vi "Color class 3 sect.vi"(7 "error in":errorcluster) -> (27 "error out":errorcluster)   [LabVIEW 2020]
uses:
  <vilib>/vision/Classification.llb/IMAQ Classifier Read Options.ctl
  <vilib>/vision/NI_Vision_Development_Module.lvlib
panel:
  out "Image Out":T1(plugin-control)
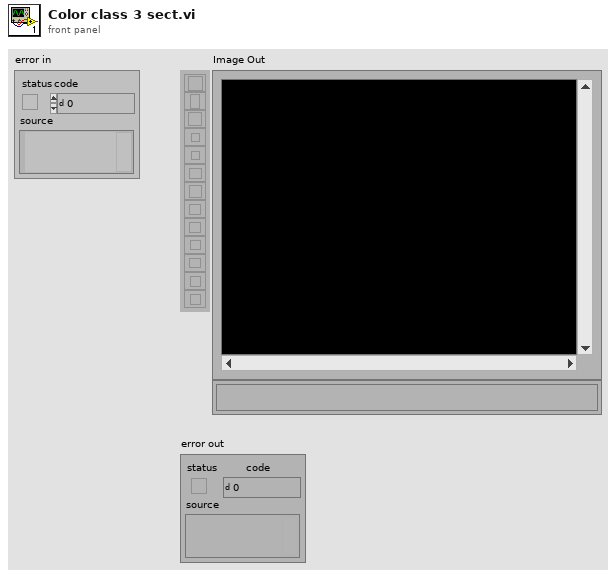
[diagram p1: front panel]
types:
  T1 = typedef "IMAQ Image.ctl" = refnum<image>
  T2 = cluster{"Global Rectangle":i32[], "Contours":cluster{"ID":enum32{"External", "Internal"}, "Type":u32, "Coordinates":i32[]}[]}
  T3 = typedef "Image Type" = u32
  T4 = typedef "IMAQ Classifier Read Options.ctl" = i32
  T5 = typedef "IMAQ Classifier Session.ctl" = refnum<k1>
  T6 = typedef "ROI Descriptor" = cluster{"Global Rectangle":i32[], "Contours":cluster{"ID":enum32{"External", "Internal"}, "Type":u32, "Coordinates":i32[]}[]}
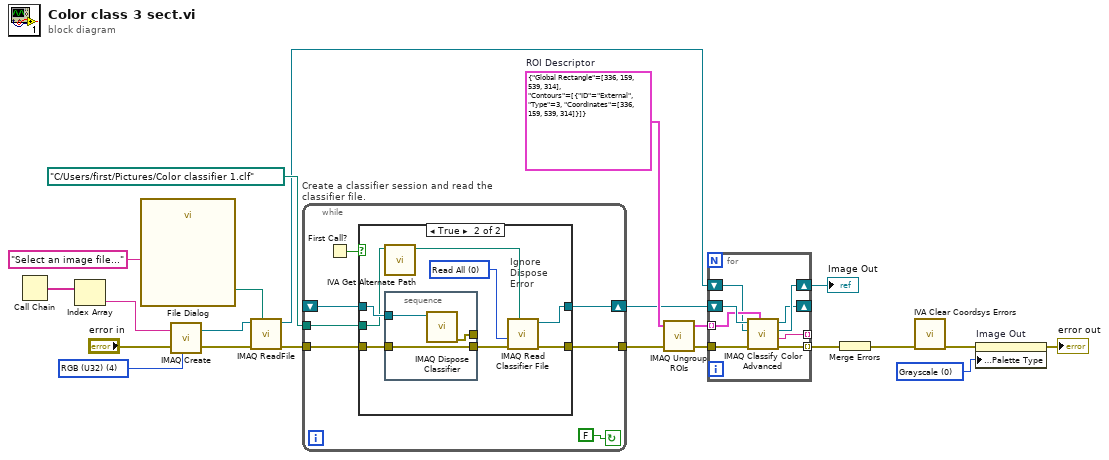
[diagram p0: block diagram]
diagram:
  w1 = u32 0 items=["Grayscale", "Binary", "Gradient", "Rainbow", "Temperature", "User Defined", "Binary 16 Bit", "Gradient 16 Bit", "Rainbow 16 Bit", "Temperature 16 Bit", "User Defined 16 Bit"] ("Palette Type")
  w13 = T2 {"Global Rectangle"=[336, 159, 539, 314], "Contours"=[{"ID"=enum."External", "Type"=3, "Coordinates"=[336, 159, 539, 314]}]}  # ROI Descriptor
  w15 = T3 4 items=["Grayscale (U8)", "Grayscale (I16)", "Grayscale (SGL)", "Complex (CSG)", "RGB (U32)", "HSL (U32)", "RGB (U64)", "Grayscale (U16)"] ("Image Type")
  n1 = Call Chain() -> (call chain=w19:string[])
  n2 = Index Array(array=w19) -> (element=w18:string)  [unwired: 1 in]
  n3 = call "File Dialog"("prompt"="Select an image file...") -> ("selected path"=w16:path)  [unwired: 6 in, 8 out]
  n4 = call "IMAQ Create"("Image Name"=w18, "Image Type"=w15, "error in (no error)"="error in") -> ("New Image"=w22:T1, "error out"=w21:errorcluster)  [unwired: 1 in, 1 out]
  n5 = call "IMAQ ReadFile"("File Path"=w16, "error in (no error)"=w21, "Image"=w22) -> ("error out"=w12:errorcluster, "Image Out"=w6:T1)  [unwired: 2 in, 5 out]
  n6 = while "Create a classifier session and read the classifier file." {
    shift-right: [w29] -> w5
    shift-left: _ -> [w28]
    tunnel: w12 -> [w26]
    tunnel: [w25] -> w11
    tunnel: path "C:/Users/first/Pictures/Color classifier 1.clf" ("File Path") -> [w24]
    stop <- FALSE continue-if-true
    n7 = First Call?() -> (First Call?: T/F=w23:bool)
    n8 = case shown="True" w23 {
      tunnel: [w31 w38] -> w29
      tunnel: w28 -> [w31 w36]
      tunnel: w26 -> [w30 w35]
      tunnel: [w30 w37] -> w25
      tunnel: w24 -> [_ w33]
      frame False {
      }
      frame True {
        w39 = T4 0 items=["Read All", "Add Samples, Do Not Change Options", "Read Options, Do Not Add Samples"] ("Read Options")
        # "Ignore Dispose Error"
        n9 = call <vilib>:"IVA Get Alternate Path.vi"("Path In"=w33) -> ("Path Out"=w32:path)  [unwired: 10 out]
        n10 = stacked-sequence {
          tunnel: w36 -> [w42]
          tunnel: w35 -> [w41]
          tunnel: [w41] -> w34
          tunnel: [w40] -> _
          frame #0 {
            n11 = call "IMAQ Dispose Classifier"("Classifier Session"=w42) -> ("error out"=w40:errorcluster)  [unwired: 1 in, 9 out]
          }
        }
        n12 = call "IMAQ Read Classifier File"("File Path"=w32, "error in (no error)"=w34, "Read Options"=w39) -> ("error out"=w37:errorcluster, "Classifier Session"=w38:T5)  [unwired: 1 in, 6 out]
      }
    }
  }
  n13 = call "IMAQ Ungroup ROIs"("error in (no error)"=w11, "ROI Descriptor"=w13) -> ("error out"=w10:errorcluster, "ROI Descriptors out"=w9:T6[])  [unwired: 2 out]
  n14 = for {
    tunnel: [w50] -> _ mode=indexing
    tunnel: [w49] -> w8 mode=indexing
    tunnel: w10 -> [w47]
    tunnel: w9 -> [w46] mode=indexing
    shift-right: [w44] -> w2
    shift-left: w6 -> [w45]
    shift-right: [w43] -> _
    shift-left: w5 -> [w48]
    n15 = call "IMAQ Classify Color Advanced"("ROI Descriptor"=w46, "error in (no error)"=w47, "Image"=w45, "Classifier Session"=w48) -> ("error out"=w49:errorcluster, "Class"=w50:string, "Image (dup)"=w44:T1, "Classifier Session (dup)"=w43:T5)  [unwired: 4 out]
  }
  "Image Out" <- w2
  n16 = Merge Errors(w8) -> (w7:errorcluster)
  n17 = call <vilib>:"IVA Clear Coordsys Errors.vi"("error in (no error)"=w7) -> ("error out"=w4:errorcluster)  [unwired: 10 in]
  n18 = property on="Image Out" class="ImageControl"(error in=w4, "Palette:Palette Type"=w1) -> (error out=→"error out":errorcluster)  [unwired: 1 in, 1 out]
